vi "SEQUSE~1.VI"(5 "testConfigCluster":T2={"slotIndex"=0, "execMode"=enum."Run", "mainConfigFile"=path "", "criteriaINI"=path "", "totalResult"=FALSE, "stopIfFail"=TRUE, "userControls"={"dialog"=refnum, "testTable"=refnum, "stopButton"=refnum, "statusBox"=refnum}, "testedResult"=enum."DONE", "timeStamp"={"Start"=timestamp(0 s since 1904-01-01), "End"=timestamp(0 s since 1904-01-01)}, "repeatNum"=1, "uutInfo"={"s/n"="", "p/n"="", "productRev"=""}, "sysLanguage"=enum."English", "numOfSocket#"=1, "testRef"="", "testInfo"={"testTime"="", "userID"="", "stationName"="", "testerID"="", "hwVer"="", "swVer"="", "fixtureID"=""}} caption="testConfigCluster (DO NOT REMOVE)", 7 "seqProperties":T1={"Properties"={"processModel"=enum."Single Test", "callSetup"=enum."One-time only when load sequence", "snSetting"={"RequireSnScan?"=TRUE, "digits"=-1.0, "regExp"="", "fixedBarcodeScannerPath"=path ""}, "stopIfFail?"=TRUE, "retestConfirm?"=TRUE, "numTestSocket"=1}, "productInfo"={"Name"="", "Pn"="", "parameter"=variant, "ProdVer"="", "hwVer"="", "swVer"="", "stationName"="", "testerNumber"="1", "fixtureID"=""}, "path"={"criteriaINIPath"=path ""}} caption="seqProperties (DO NOT REMOVE)", 8 "errorIn":errorcluster, 9 "Result?":bool, 11 "sysVar":T4 caption="sysVar (DO NOT REMOVE)") -> (0 "error out":errorcluster, 3 "createLogSuccesful":bool caption="Create Log Succesful (DO NOT REMOVE)")   [LabVIEW 2020]
uses:
  <userlib>/_ATMF/Control_Typedef/__ATMF__SYSTEM__VARIABLE__.ctl
  <userlib>/_ATMF/Control_Typedef/__SEQ__REFERENCE__VARIABLES__.ctl
  <userlib>/_ATMF/Control_Typedef/__SEQ__SYSTEM__CONFIG__UI__USER__DEFINITION__VARIABLES__.ctl
  <userlib>/_ATMF/Tools/Control/__TEST__SEQ__CONFIG__CLUSTER__.ctl
  <userlib>/_ATMF/Control_Typedef/__TEST__STEP__VAR__UI__EXEC__MODE__.ctl
  <userlib>/_ATMF/Control_Typedef/__ATMF__MAIN__TEST__SEQ__PROPERTIES__.ctl
  <vilib>/Comparison/Equal/Equal Functor/Equal Functor.lvclass
panel:
  out "sysVar(Duplicated)":T4
  # "( -1 mean skip check)"
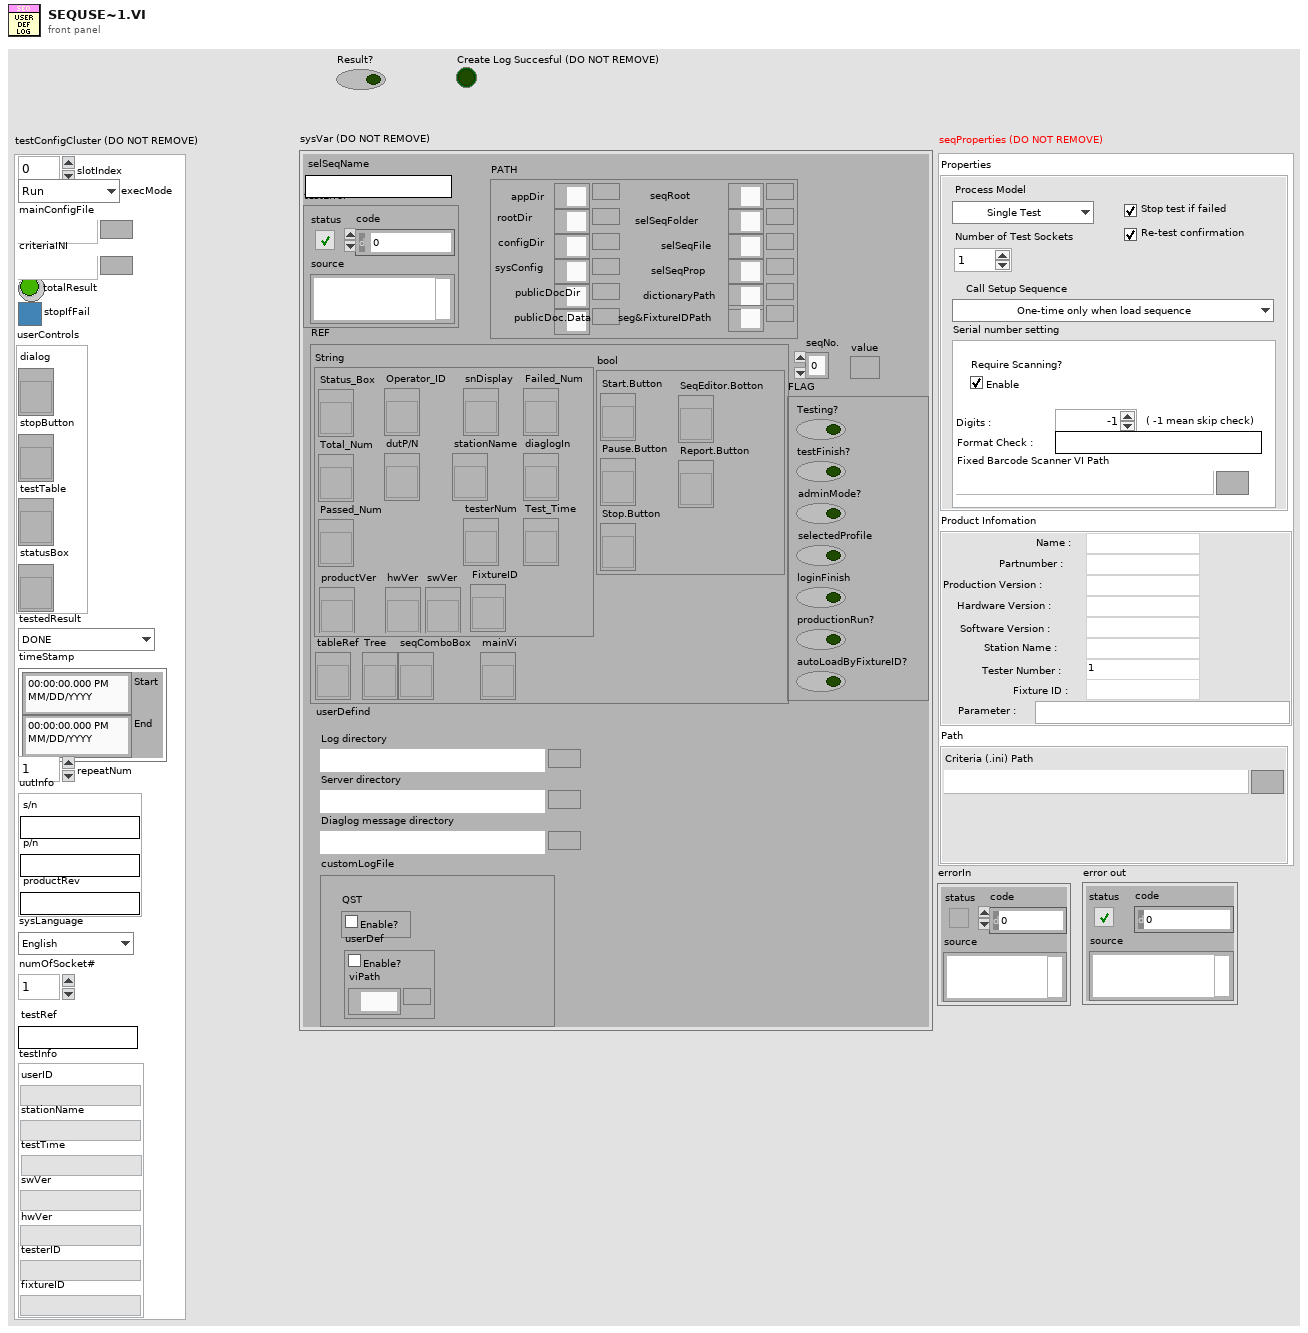
[diagram p1: front panel]
types:
  T1 = typedef "__ATMF__MAIN__TEST__SEQ__PROPERTIES__.ctl" = cluster{"Properties":cluster{"processModel":enum16{"Single Test", "Batch Test", "Parallel Test"}, "callSetup":enum16{"Every test loop", "One-time only when load sequence"}, "snSetting":cluster{"RequireSnScan?":bool, "digits":dbl, "regExp":string, "fixedBarcodeScannerPath":path}, "stopIfFail?":bool, "retestConfirm?":bool, "numTestSocket":u8}, "productInfo":cluster{"Name":string, "Pn":string, "parameter":variant, "ProdVer":string, "hwVer":string, "swVer":string, "stationName":string, "testerNumber":string, "fixtureID":string}, "path":cluster{"criteriaINIPath":path}}
  T2 = typedef "__TEST__SEQ__CONFIG__CLUSTER__.ctl" = cluster{"slotIndex":u8, "execMode":T3, "mainConfigFile":path, "criteriaINI":path, "totalResult":bool, "stopIfFail":bool, "userControls":cluster{"dialog":refnum<vi>, "testTable":refnum<vi>, "stopButton":refnum<vi>, "statusBox":refnum<vi>}, "testedResult":enum16{"DONE", "PASS", "FAIL", "ERROR", "SKIPPED"}, "timeStamp":cluster{"Start":timestamp, "End":timestamp}, "repeatNum":u8, "uutInfo":cluster{"s/n":string, "p/n":string, "productRev":string}, "sysLanguage":enum16{"English", "Chinese", "Thai"}, "numOfSocket#":u8, "testRef":string, "testInfo":cluster{"testTime":string, "userID":string, "stationName":string, "testerID":string, "hwVer":string, "swVer":string, "fixtureID":string}}
  T3 = typedef "__TEST__STEP__VAR__UI__EXEC__MODE__.ctl" = enum16{"Run", "Debug", "Edit", "Open VI"}
  T4 = typedef "__ATMF__SYSTEM__VARIABLE__.ctl" = cluster{"seqNo.":i32, "testError":errorcluster, "value":variant, "REF":T5, "PATH":cluster{"appDir":path, "rootDir":path, "configDir":path, "sysConfig":path, "publicDocDir":path, "publicDoc.Data":path, "seqRoot":path, "selSeqFolder":path, "selSeqFile":path, "selSeqProp":path, "dictionaryPath":path, "seg&FixtureIDPath":path}, "FLAG":cluster{"Testing?":bool, "testFinish?":bool, "adminMode?":bool, "selectedProfile":bool, "loginFinish":bool, "productionRun?":bool, "autoLoadByFixtureID?":bool}, "userDefind":T6, "selSeqName":string, "customLogFile":cluster{"QST":cluster{"Enable?":bool}, "userDef":cluster{"Enable?":bool, "viPath":path}}}
  T5 = typedef "__SEQ__REFERENCE__VARIABLES__.ctl" = cluster{"String":cluster{"Status_Box":refnum<vi>, "Total_Num":refnum<vi>, "Passed_Num":refnum<vi>, "Failed_Num":refnum<vi>, "diaglogIn":refnum<vi>, "Test_Time":refnum<vi>, "Operator_ID":refnum<vi>, "snDisplay":refnum<vi>, "stationName":refnum<vi>, "testerNum":refnum<vi>, "productVer":refnum<vi>, "dutP/N":refnum<vi>, "hwVer":refnum<vi>, "swVer":refnum<vi>, "FixtureID":refnum<vi>}, "bool":cluster{"SeqEditor.Botton":refnum<vi>, "Start.Button":refnum<vi>, "Pause.Button":refnum<vi>, "Stop.Button":refnum<vi>, "Report.Button":refnum<vi>}, "tableRef":refnum<vi>, "Tree":refnum<vi>, "seqComboBox":refnum<vi>, "mainVi":refnum<vi>}
  T6 = typedef "__SEQ__SYSTEM__CONFIG__UI__USER__DEFINITION__VARIABLES__.ctl" = cluster{"resultLog":path, "serverLogPath":path, "diagMsgDir":path}
  T7 = cluster{"resultArray2D[]":string[][], "createLogSuccesful":bool}
  T8 = enum16{"Reset", "Yellow Lamp&Alarm", "Green Lamp&Alarm", "Red Lamp&Alarm"}
  T9 = enum16{"Step", "Description", "Min", "Measure", "Max", "Unit", "Status"}
  T10 = enum16{"open", "replace", "create", "open or create", "replace or create", "replace or create with confirmation"}
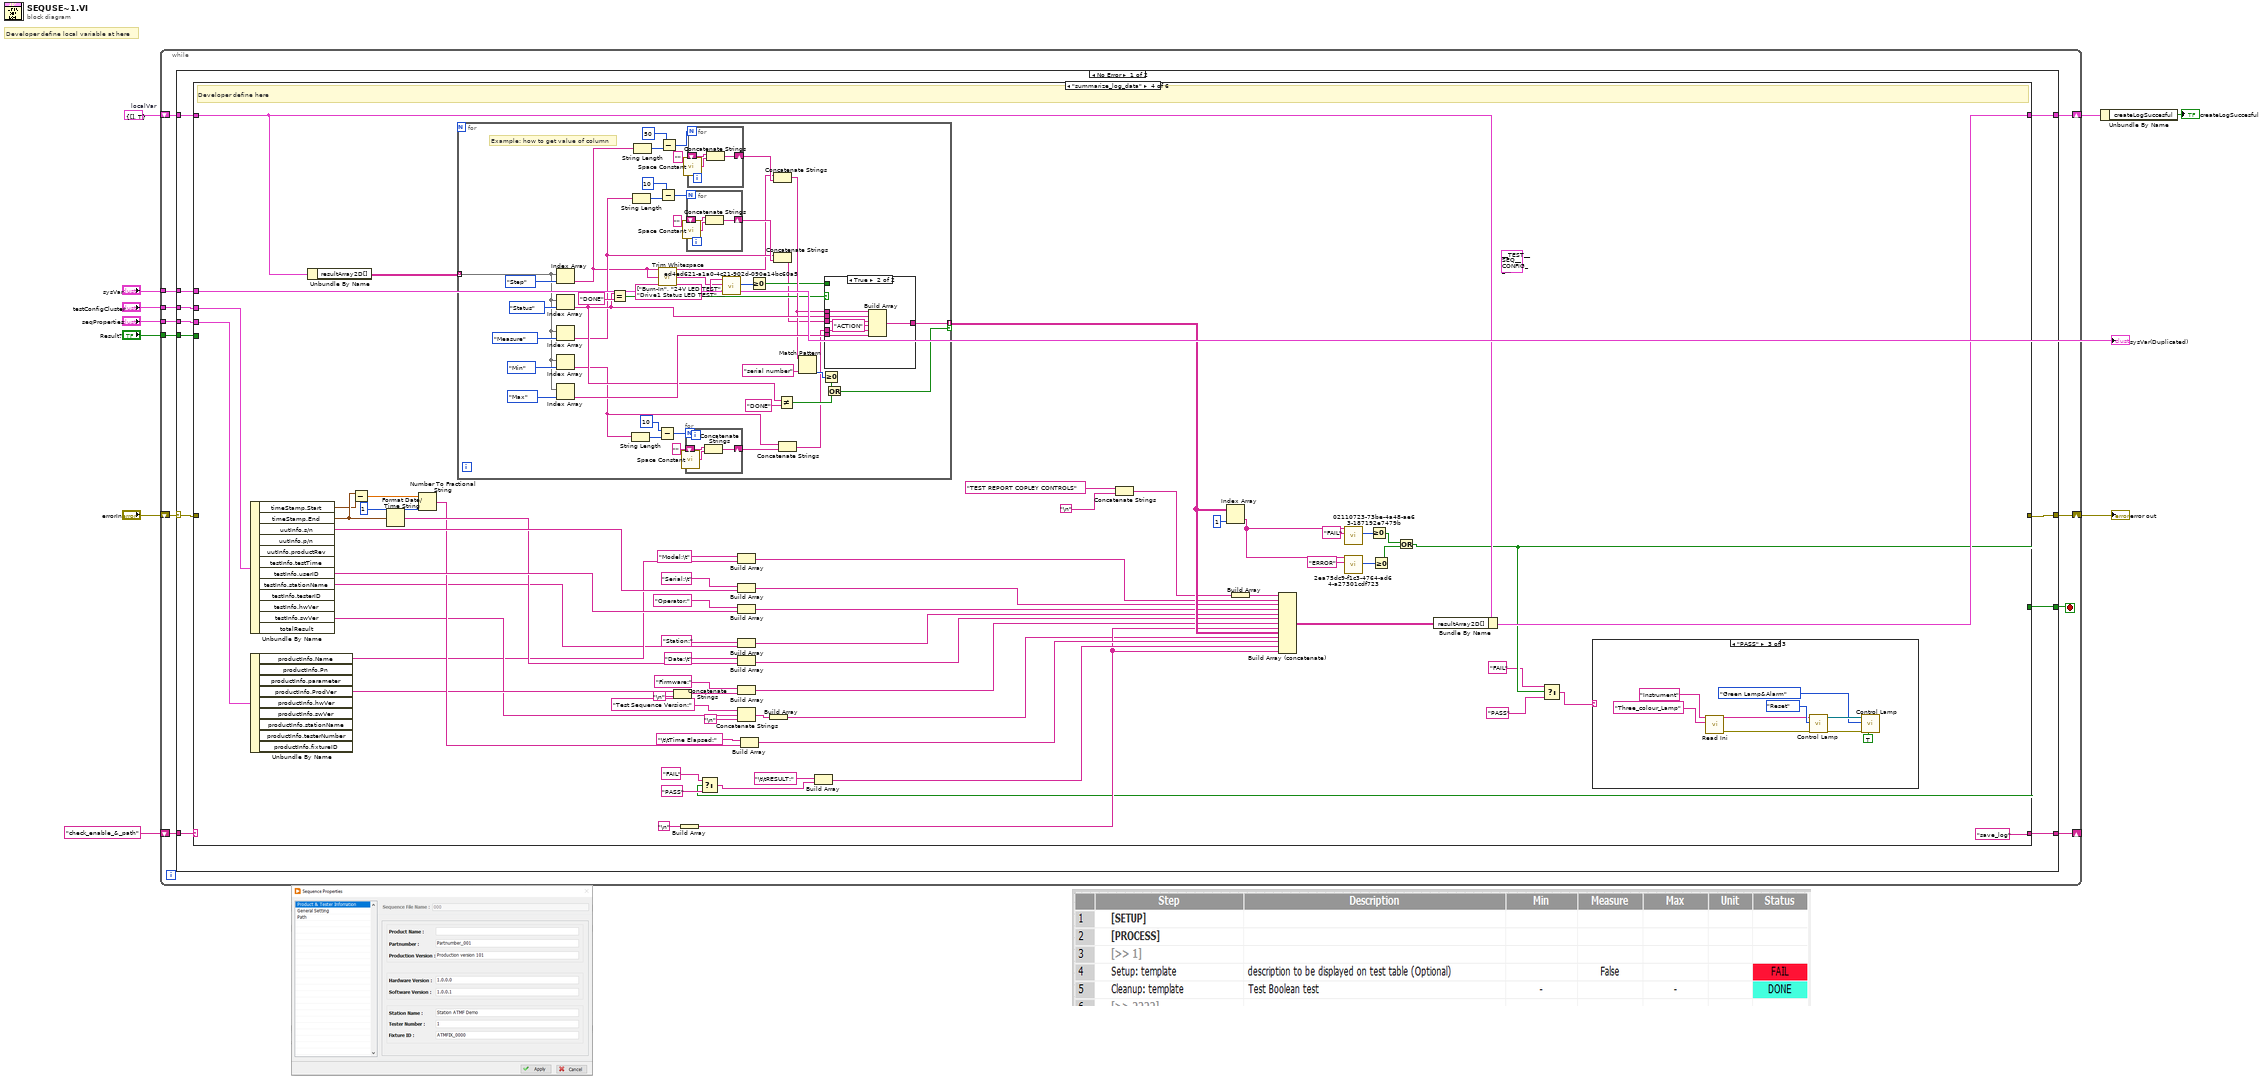
[diagram p0: block diagram]
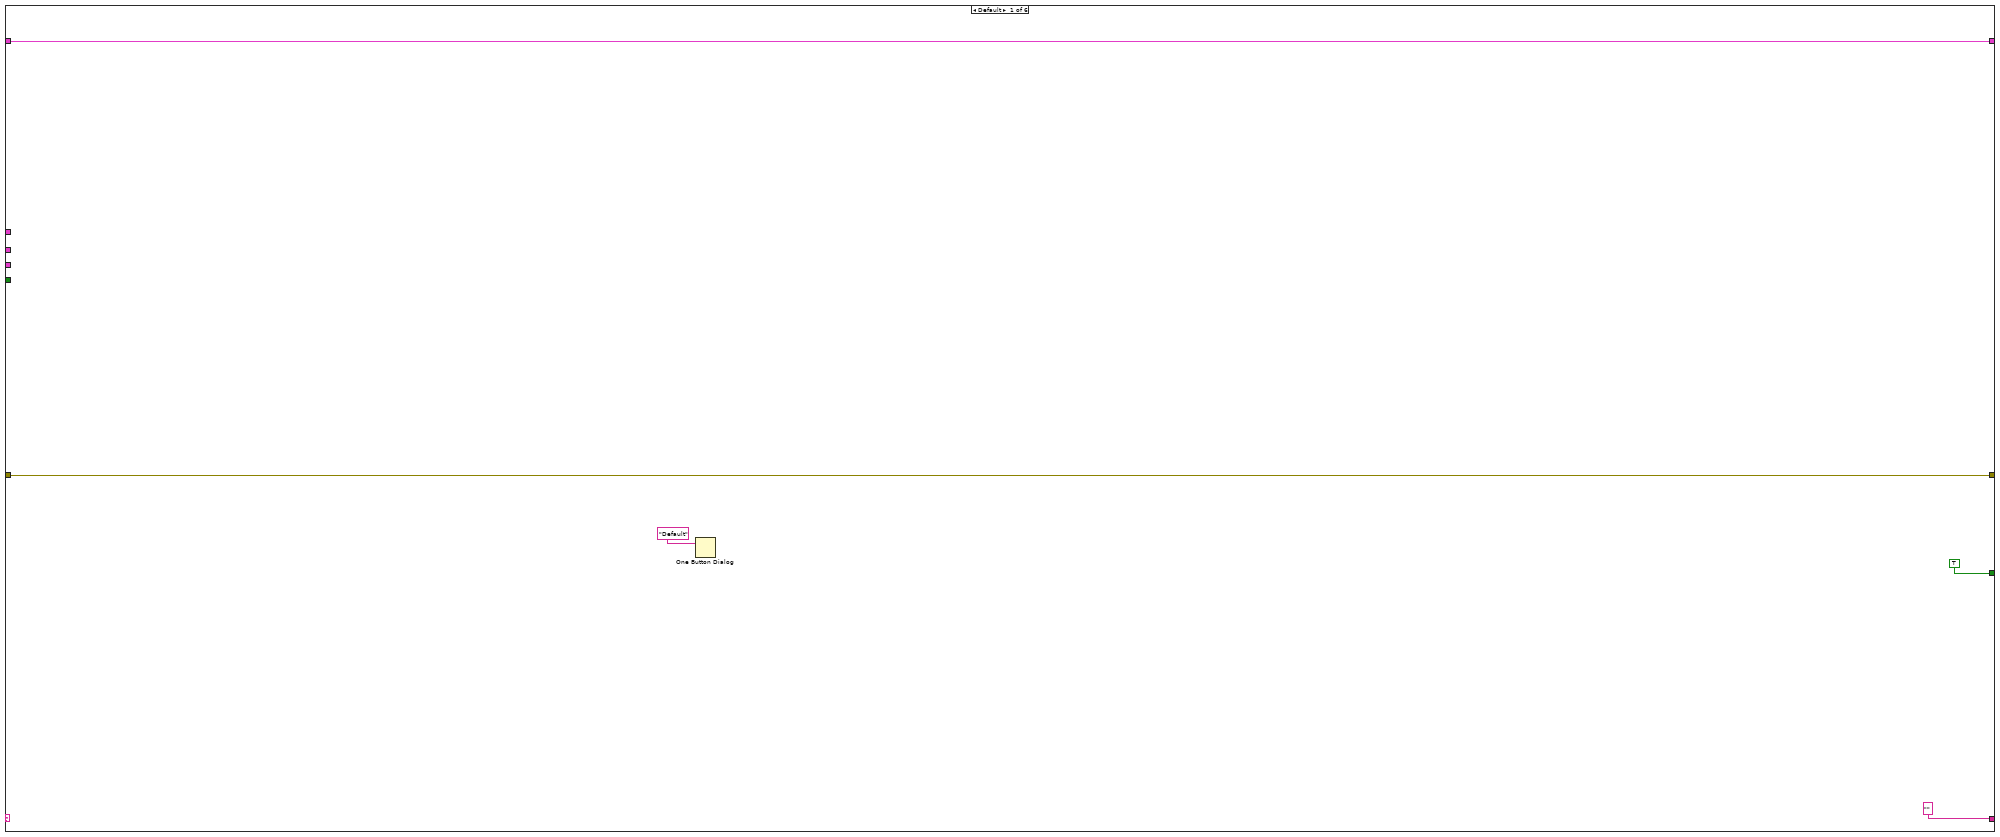
[diagram p2: hidden frame]
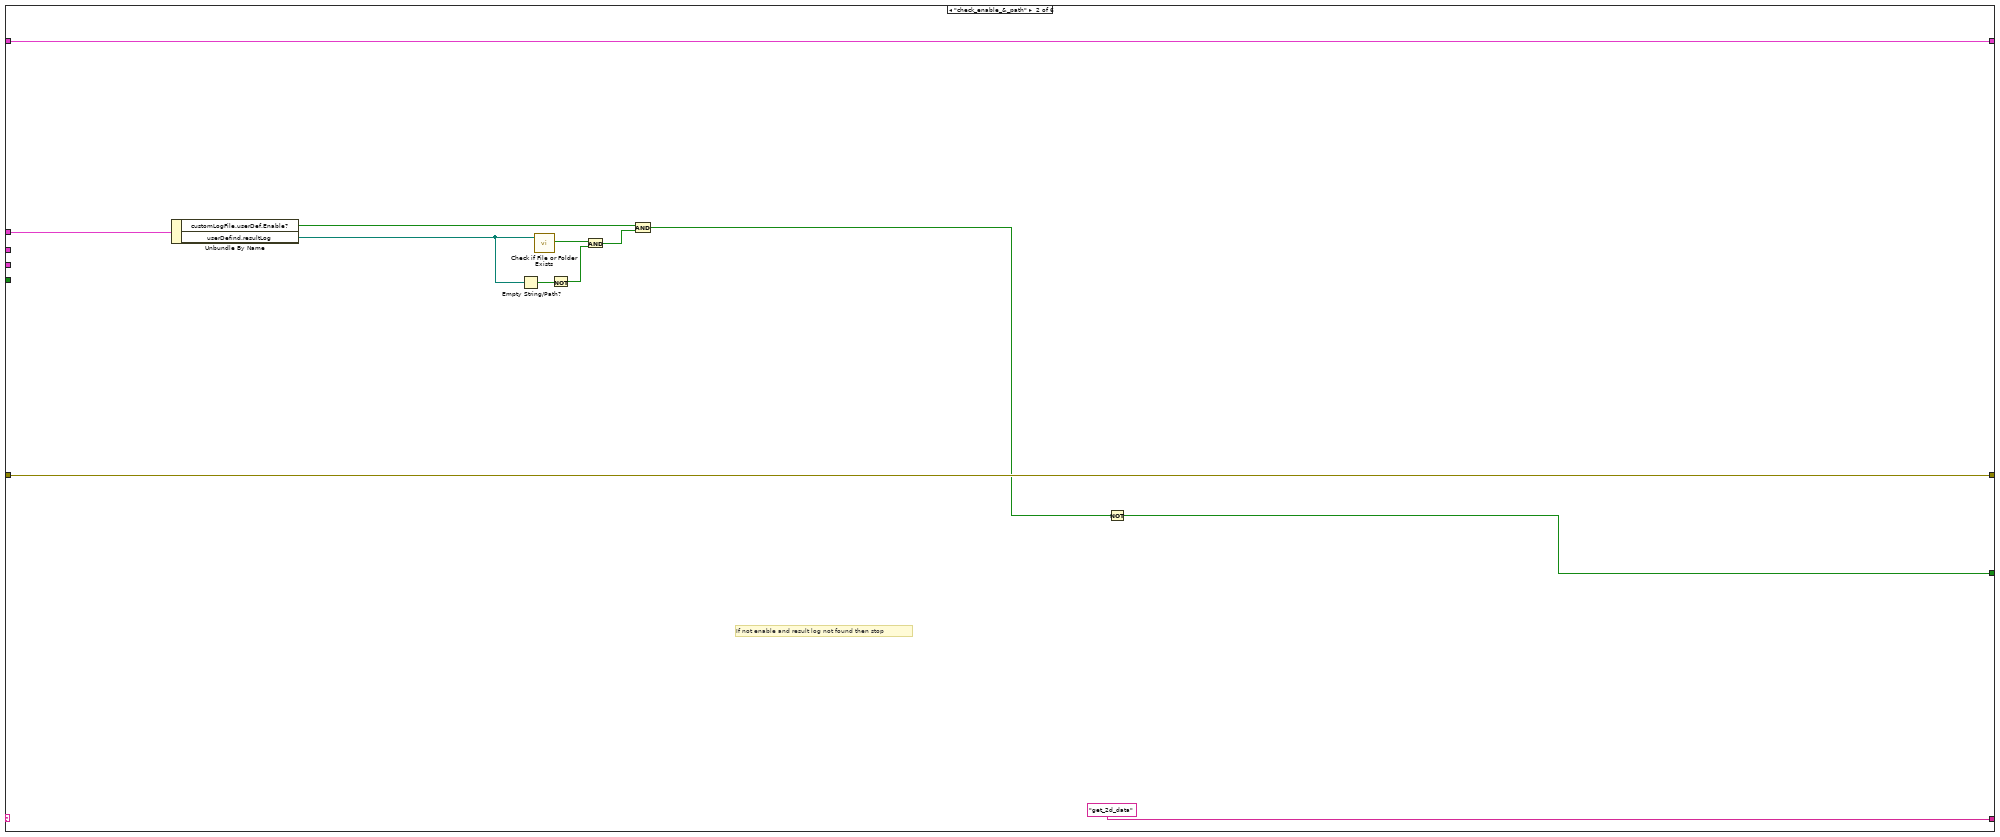
[diagram p3: hidden frame]
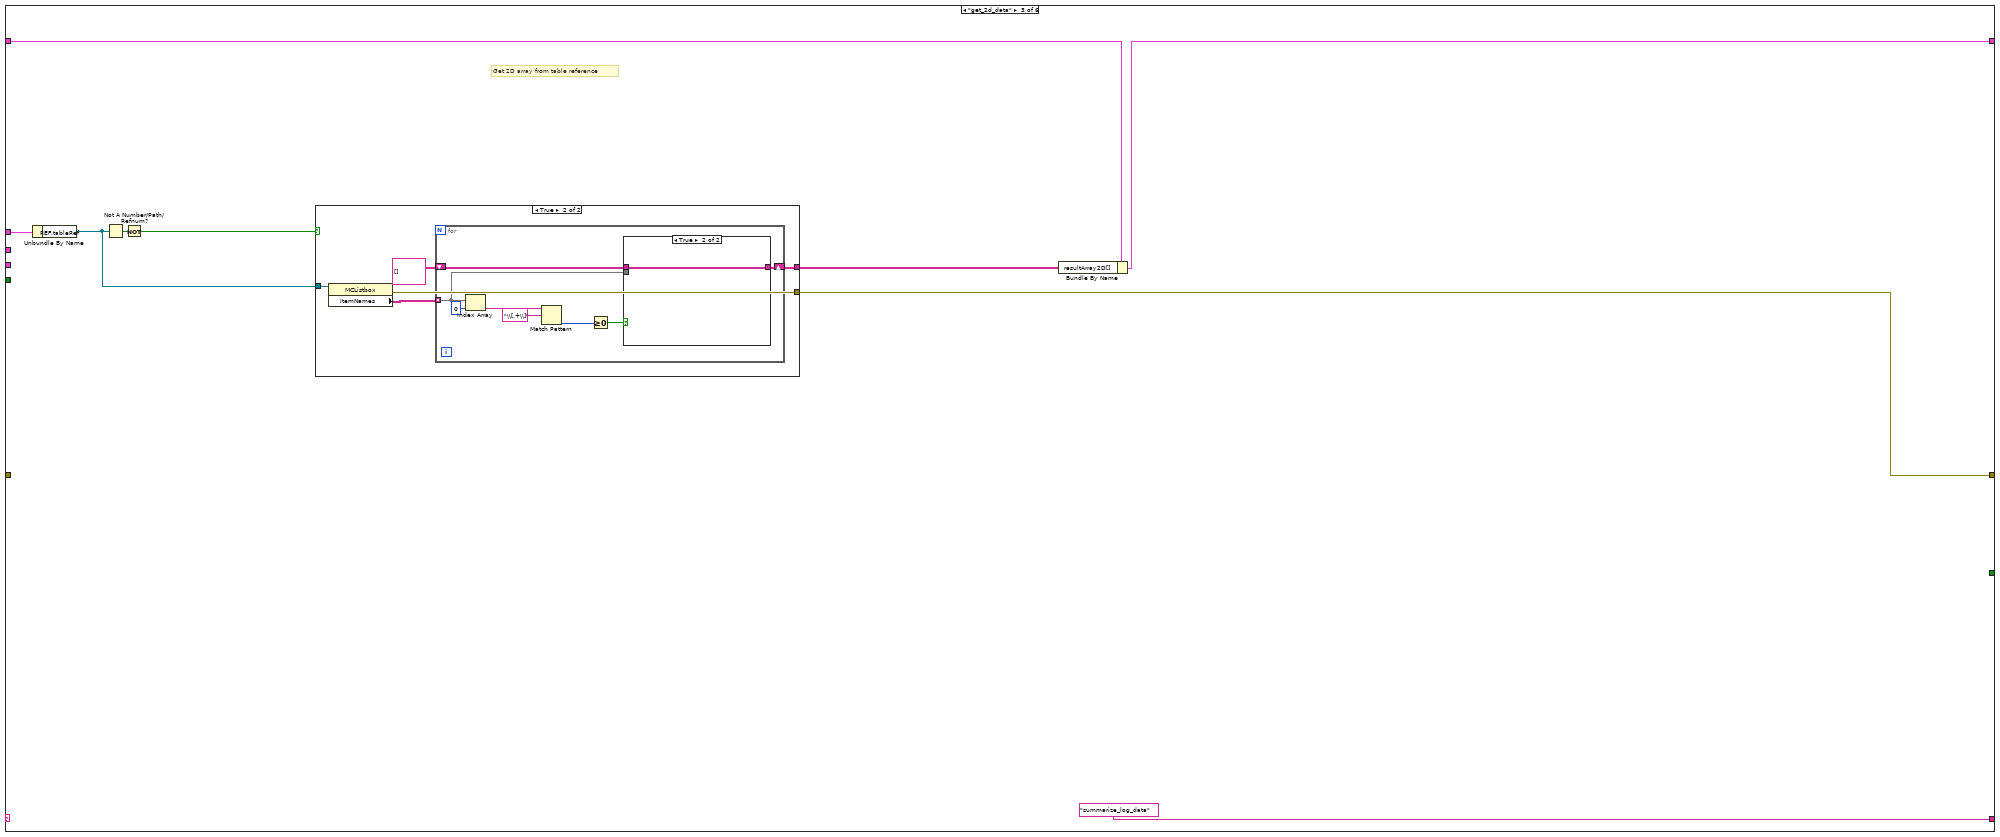
[diagram p4: hidden frame]
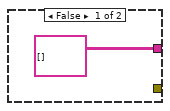
[diagram p5: hidden frame]
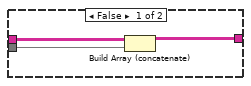
[diagram p6: hidden frame]
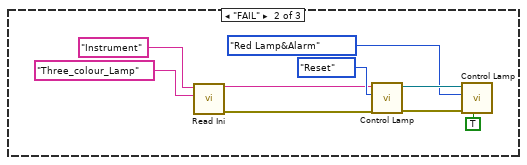
[diagram p8: hidden frame]
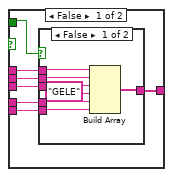
[diagram p9: hidden frame]
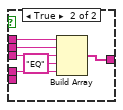
[diagram p10: hidden frame]
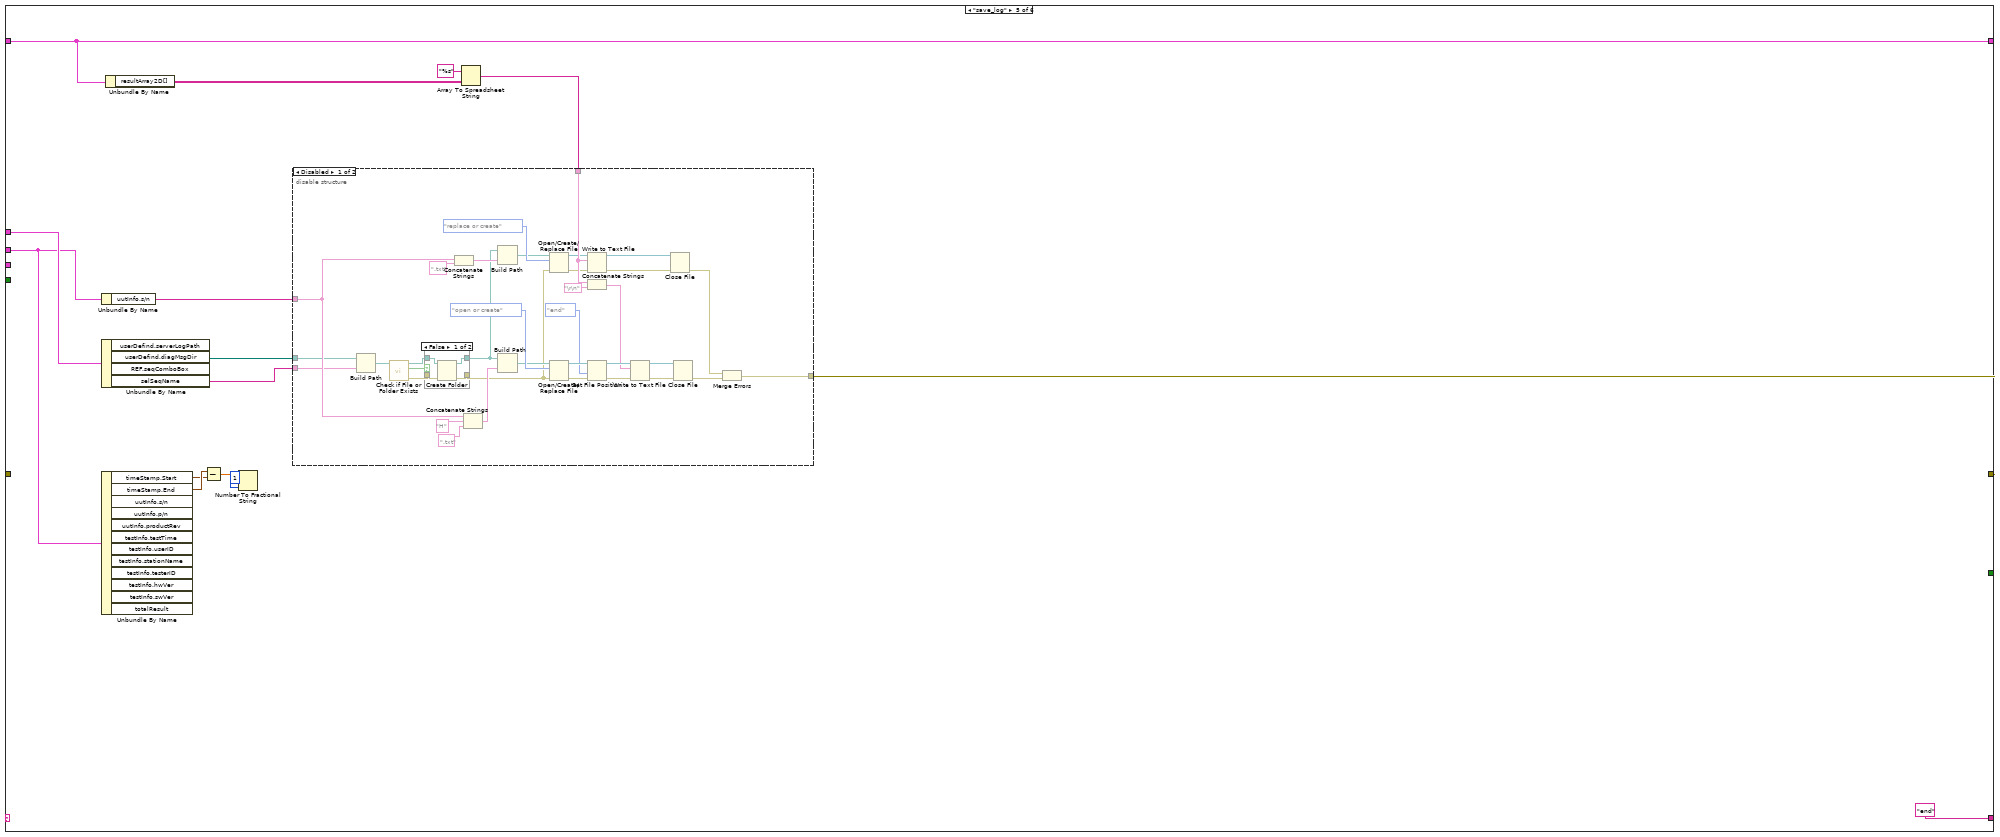
[diagram p11: hidden frame]
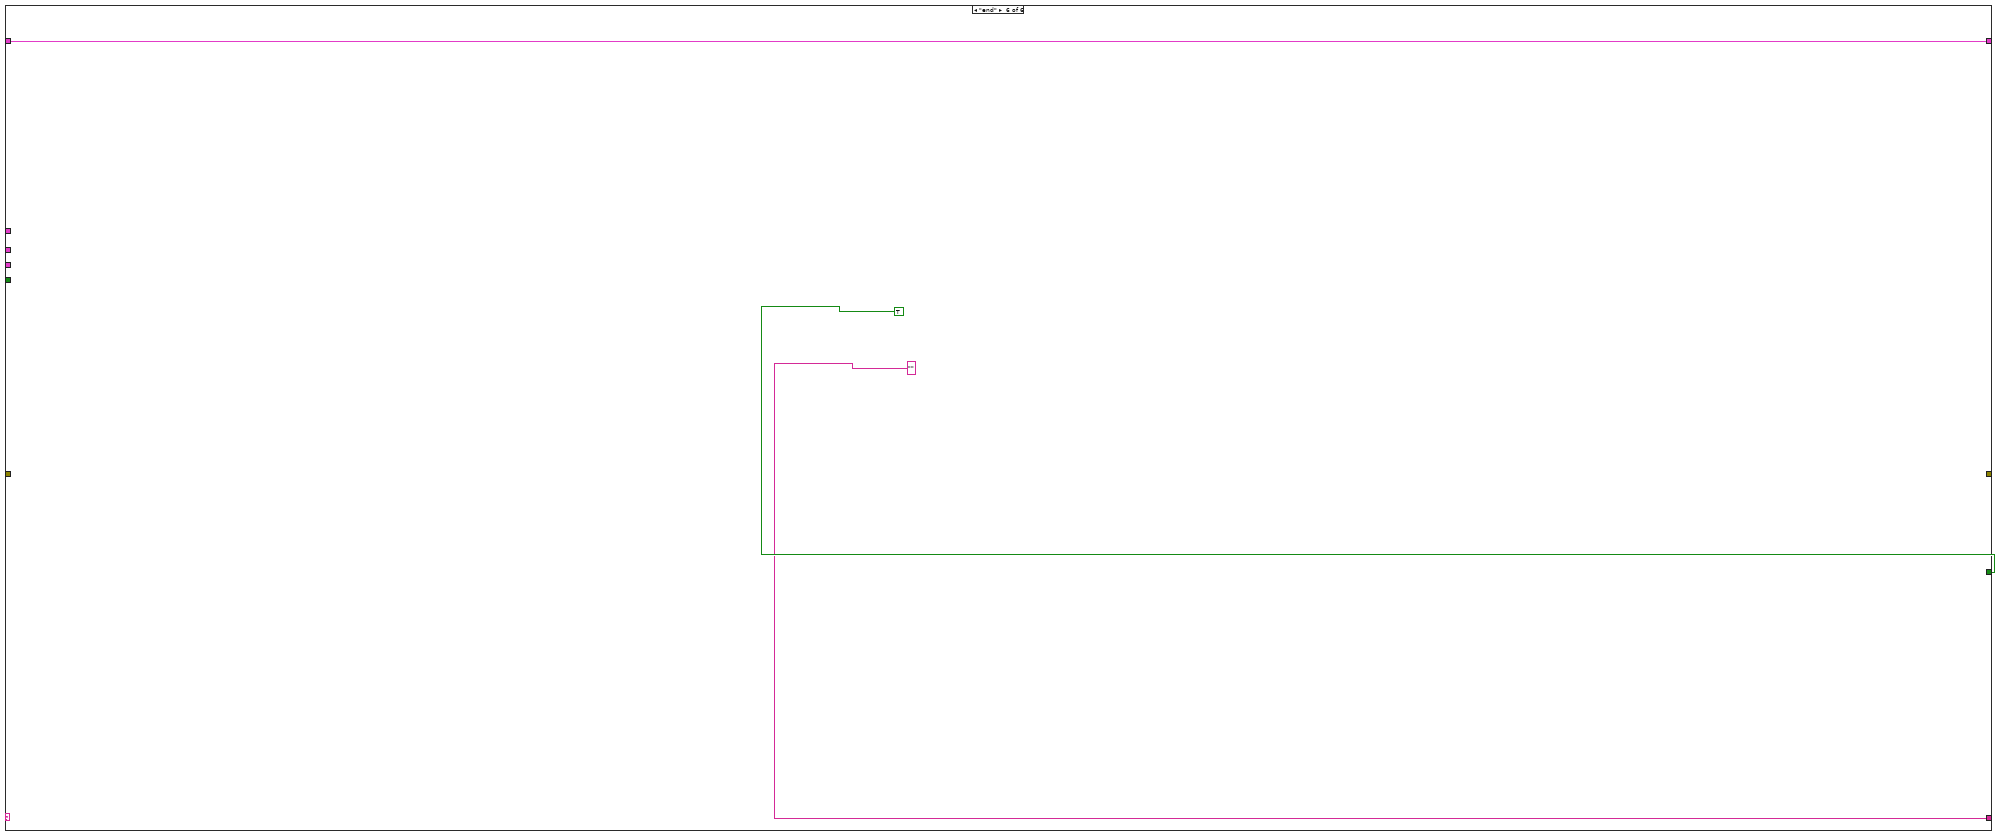
[diagram p14: hidden frame]
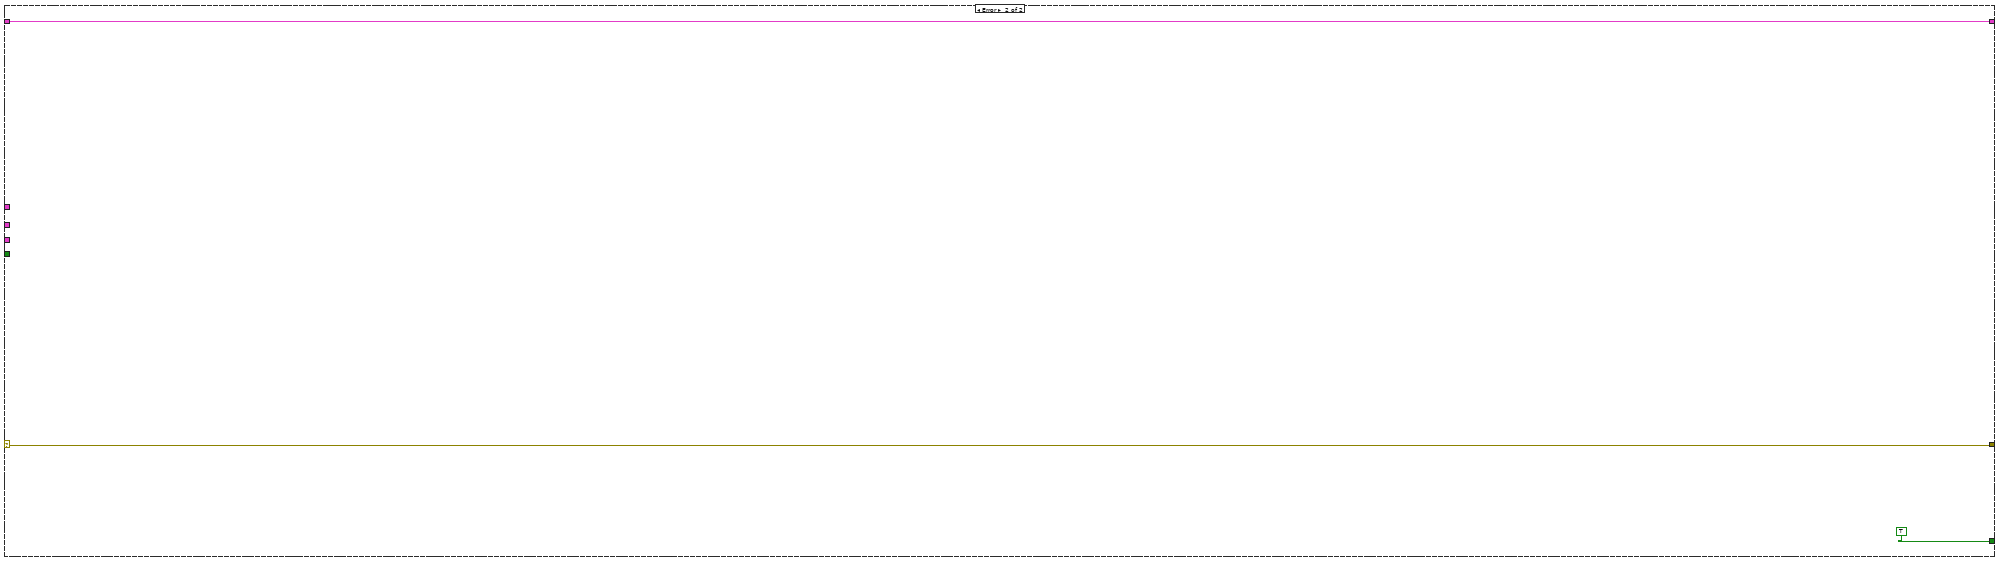
[diagram p15: hidden frame]
diagram:
  w3 = T7 {"resultArray2D[]"=[], "createLogSuccesful"=TRUE}  # localVar
  # "Developer define local variable at here"
  n1 = while {
    shift-right: [w19] -> w10
    shift-left: "errorIn" -> [w20]
    tunnel: "sysVar" -> [w17]
    tunnel: "testConfigCluster" -> [w16]
    tunnel: "seqProperties" -> [w15]
    shift-right: [w18] -> _
    shift-left: "check_enable_&_path" -> [w21]
    tunnel: "Result?" -> [w14]
    shift-right: [w11] -> w2
    shift-left: w3 -> [w12]
    stop <- w13 stop-if-true
    n2 = case shown="No Error" w20 {
      selector: w20 -> [w31 w297]
      tunnel: w21 -> [w32 _]
      tunnel: [w30 w297] -> w19
      tunnel: [w29 _] -> w18
      tunnel: w17 -> [w28 _]
      tunnel: w16 -> [w27 _]
      tunnel: w15 -> [w26 _]
      tunnel: w14 -> [w25 _]
      tunnel: [w24 TRUE] -> w13
      tunnel: w12 -> [w23 w295]
      tunnel: [w22 w295] -> w11
      frame No Error {
        n3 = case shown="\"summarize_log_data\"" w32 {
          tunnel: w31 -> [w37 w49 _ _ _ _]
          tunnel: [w37 w49 w50 _ w246 _] -> w30
          tunnel: ["" "get_2d_data" "summarize_log_data" "save_log" "end" ""] -> w29
          tunnel: w28 -> [_ w41 w58 _ w242 _]
          tunnel: w27 -> [_ _ _ w85 w236 _]
          tunnel: w26 -> [_ _ _ w88 _ _]
          tunnel: w25 -> [_ _ _ _ _ _]
          tunnel: [TRUE w39 _ _ _ TRUE] -> w24
          tunnel: w23 -> [w34 w38 w54 w138 w249 w294]
          tunnel: [w34 w38 w53 w92 w249 w294] -> w22
          frame Default {
            n4 = One Button Dialog(message="Default") -> ()  [unwired: 1 in, 1 out]
          }
          frame "check_enable_&_path" {
            # "If not enable and result log not found then stop"
            n5 = Unbundle By Name(w41) -> ("customLogFile.userDef.Enable?"=w42:bool, "userDefind.resultLog"=w46:path)
            n6 = Empty String/Path?(string/path=w46) -> (empty?=w43:bool)
            n7 = call <vilib>:"Check if File or Folder Exists.vi"("path"=w46) -> ("file or folder exists?"=w44:bool)  [unwired: 8 in, 2 out]
            n8 = Not(x=w43) -> (.not. x?=w45:bool)
            n9 = And(x=w44, y=w45) -> (x .and. y?=w47:bool)
            n10 = And(x=w42, y=w47) -> (x .and. y?=w40:bool)
            n11 = Not(x=w40) -> (.not. x?=w39:bool)
          }
          frame "get_2d_data" {
            # "Get 2D array from table reference"
            n12 = Unbundle By Name(w58) -> ("REF.tableRef"=w55:refnum<vi>)
            n13 = Not A Number/Path/Refnum?(number/path/refnum=w55) -> (NaN/Path/Refnum?=w57:bool)
            n14 = Not(x=w57) -> (.not. x?=w56:bool)
            n15 = case shown="True" w56 {
              tunnel: [string[][] [] w62] -> w52
              tunnel: w55 -> [_ w61]
              tunnel: [_ w60] -> w50
              frame False {
              }
              frame True {
                n16 = property class="MCListbox"(reference=w61) -> (error out=w60:errorcluster, "ItemNames"=w64:string[][])  [unwired: 1 in, 1 out]
                n17 = for {
                  tunnel: w64 -> [w65] mode=indexing
                  shift-right: [w68] -> w62
                  shift-left: string[][] [] -> [w69]
                  n18 = Index Array(array=w65, index=0) -> (element=w71:string)
                  n19 = Match Pattern(string=w71, regular expression="\\[.+\\]") -> (offset past match=w67:i32)  [unwired: 1 in, 3 out]
                  n20 = Greater Or Equal To 0?(x=w67) -> (x >= 0?=w66:bool)
                  n21 = case shown="True" w66 {
                    tunnel: w69 -> [w75 w76]
                    tunnel: [w74 w76] -> w68
                    tunnel: w65 -> [w73 _]
                    frame False {
                      n22 = Build Array (concatenate)(w75, w73) -> (w74:string[][])
                    }
                    frame True {
                    }
                  }
                }
              }
            }
            n23 = Bundle By Name(cluster=w54, "resultArray2D[]"=w52) -> (w53:T7)
          }
          frame "summarize_log_data" {
            (unwired) T2 {"slotIndex"=0, "execMode"=enum."Run", "mainConfigFile"=path "", "criteriaINI"=path "", "totalResult"=FALSE, "stopIfFail"=FALSE, "userControls"={"dialog"=refnum, "testTable"=refnum, "stopButton"=refnum, "statusBox"=refnum}, "testedResult"=enum."DONE", "timeStamp"={"Start"=timestamp(0 s since 1904-01-01), "End"=timestamp(0 s since 1904-01-01)}, "repeatNum"=1, "uutInfo"={"s/n"="", "p/n"="", "productRev"=""}, "sysLanguage"=enum."English", "numOfSocket#"=1, "testRef"="", "testInfo"={"testTime"="", "userID"="", "stationName"="", "testerID"="", "hwVer"="", "swVer"="", "fixtureID"=""}} ("testConfigCluster")
            # "Developer define here"
            n24 = Unbundle By Name(w85) -> ("timeStamp.Start"=w120:timestamp, "timeStamp.End"=w121:timestamp, "uutInfo.s/n"=w135:string, "testInfo.userID"=w133:string, "testInfo.stationName"=w83:string, "testInfo.swVer"=w94:string)  [unwired: 6 out]
            n25 = Unbundle By Name(w88) -> ("productInfo.Name"=w84:string, "productInfo.ProdVer"=w98:string)  [unwired: 7 out]
            n26 = Unbundle By Name(w138) -> ("resultArray2D[]"=w86:string[][])
            n27 = Subtract(x=w121, y=w120) -> (x-y=w119:dbl)
            n28 = Format Date/Time String(seconds (now)=w121) -> (date/time string=w130:string)  [unwired: 2 in]
            n29 = Number To Fractional String(number=w119, precision (6)=i16 1) -> (F-format string=w117:string)  [unwired: 2 in]
            n30 = for {
              tunnel: w86 -> [w179] mode=indexing
              tunnel: [w193] -> w116 mode=indexing if=w186
              # "Example: how to get value of column"
              n31 = Index Array(array=w179, index=T9."Step") -> (element=w166:string)
              n32 = Index Array(array=w179, index=T9."Status") -> (element=w185:string)
              n33 = Index Array(array=w179, index=T9."Measure") -> (element=w169:string)
              n34 = Index Array(array=w179, index=T9."Min") -> (element=w159:string)
              n35 = Index Array(array=w179, index=T9."Max") -> (element=w194:string)
              n36 = Equal?(x=w185, y="DONE") -> (x = y?=w176:bool)
              n37 = String Length(string=w159) -> (length=w162:i32)
              n38 = String Length(string=w169) -> (length=w171:i32)
              n39 = String Length(string=w166) -> (length=w184:i32)
              n40 = Subtract(x=10, y=w162) -> (x-y=w163:i32)
              n41 = call <vilib>:"Trim Whitespace.vi"("string"=w166) -> ("trimmed string"=w165:string)  [unwired: 1 in]
              n42 = Subtract(x=10, y=w171) -> (x-y=w173:i32)
              n43 = Subtract(x=50, y=w184) -> (x-y=w182:i32)
              n44 = for {
                N: w163 -> [_]
                shift-right: [w202] -> w160
                shift-left: "" -> [w201]
                n45 = call <vilib>:"Space Constant.vi"() -> ("String"=w200:string)
                n46 = Concatenate Strings(w201, w200) -> (w202:string)
              }
              n47 = for {
                N: w173 -> [_]
                shift-right: [w205] -> w170
                shift-left: "" -> [w204]
                n48 = call <vilib>:"Space Constant.vi"() -> ("String"=w203:string)
                n49 = Concatenate Strings(w204, w203) -> (w205:string)
              }
              n50 = for {
                N: w182 -> [_]
                shift-right: [w235] -> w180
                shift-left: "" -> [w234]
                n51 = call <vilib>:"Space Constant.vi"() -> ("String"=w233:string)
                n52 = Concatenate Strings(w234, w233) -> (w235:string)
              }
              n53 = call "ed4ed621-a1a0-4c21-902d-090e14bc60a5.vi"("element"=w165, "unsorted 1D array"=string[] ["Burn-In", "24V LED TEST", "Drive1 Status LED TEST", "Drive2 Status LED TEST", "Drive3 Status LED TEST", "Fan1 Test", "Fan2 Test", "Fan3 Test", "Get drive1 serial number", "Get drive2 serial number", "Get drive3 serial number", "Drive1 model number check", "Drive2 model number check", "Drive3 model number check", "Drive1 firmware version check", "Drive2 firmware version check", "Drive3 firmware version check", "Fault1 Monitor_Coil1_AMPPROG1_0V", "Fault1 Monitor_Coil1_AMPPROG1_2.5V", "Fault1 Monitor_Coil1_AMPPROG1_5V", "LED Test_the fault of M1 drive", "Fault1 Monitor_M1 Drive Fault Signal", "LED Test_Reset Drive", "Fault1 Monitor_Reset Drive", "Fault2 Monitor_Coil2_AMPPROG2_0V", "Fault2 Monitor_Coil2_AMPPROG2_2.5V", "Fault2 Monitor_Coil2_AMPPROG2_5V", "LED Test_the fault of M1 drive", "Fault2 Monitor_M1 Drive Fault Signal", "LED Test_Reset Drive", "Fault2 Monitor_Reset Drive", "Fault3 Monitor_Coil3_AMPPROG3_0V", "Fault3 Monitor_Coil3_AMPPROG3_2.5V", "Fault3 Monitor_Coil3_AMPPROG3_5V", "LED Test_the fault of M1 drive", "Fault3 Monitor_M1 Drive Fault Signal", "LED Test_Reset Drive", "Fault3 Monitor_Reset Drive", "Fault4 Monitor_Coil4_AMPPROG4_0V", "Fault4 Monitor_Coil4_AMPPROG4_2.5V", "Fault4 Monitor_Coil4_AMPPROG4_5V", "LED Test_the fault of M1 drive", "Fault4 Monitor_M1 Drive Fault Signal", "LED Test_Reset Drive", "Fault4 Monitor_Reset Drive", "Fault5 Monitor_Coil5_AMPPROG5_0V", "Fault5 Monitor_Coil5_AMPPROG5_2.5V", "Fault5 Monitor_Coil5_AMPPROG5_5V", "LED Test_the fault of M2 drive", "Fault5 Monitor_M2 Drive Fault Signal", "LED Test_Reset Drive", "Fault5 Monitor_Reset Drive", "Fault6 Monitor_Coil6_AMPPROG6_0V", "Fault6 Monitor_Coil6_AMPPROG6_2.5V", "Fault6 Monitor_Coil6_AMPPROG6_5V", "LED Test_the fault of M2 drive", "Fault6 Monitor_M2 Drive Fault Signal", "LED Test_Reset Drive", "Fault6 Monitor_Reset Drive", "Fault7 Monitor_Coil7_AMPPROG7_0V", "Fault7 Monitor_Coil7_AMPPROG7_2.5V", "Fault7 Monitor_Coil7_AMPPROG7_5V", "LED Test_the fault of M2 drive", "Fault7 Monitor_M2 Drive Fault Signal", "LED Test_Reset Drive", "Fault7 Monitor_Reset Drive", "Fault8 Monitor_Coil8_AMPPROG8_0V", "Fault8 Monitor_Coil8_AMPPROG8_2.5V", "Fault8 Monitor_Coil8_AMPPROG8_5V", "LED Test_the fault of M2 drive", "Fault8 Monitor_M2 Drive Fault Signal", "LED Test_Reset Drive", "Fault8 Monitor_Reset Drive", "Fault9 Monitor_Coil9_AMPPROG9_0V", "Fault9 Monitor_Coil9_AMPPROG9_2.5V", "Fault9 Monitor_Coil9_AMPPROG9_5V", "LED Test_the fault of M3 drive", "Fault9 Monitor_M3 Drive Fault Signal", "LED Test_Reset Drive", "Fault9 Monitor_Reset Drive", "Fault10 Monitor_Coil10_AMPPROG10_0V", "Fault10 Monitor_Coil10_AMPPROG10_2.5V", "Fault10 Monitor_Coil10_AMPPROG10_5V", "LED Test_the fault of M3 drive", "Fault10 Monitor_M3 Drive Fault Signal", "LED Test_Reset Drive", "Fault10 Monitor_Reset Drive", "Fault11 Monitor_Coil11_AMPPROG11_0V", "Fault11 Monitor_Coil11_AMPPROG11_2.5V", "Fault11 Monitor_Coil11_AMPPROG11_5V", "LED Test_the fault of M3 drive", "Fault11 Monitor_M3 Drive Fault Signal", "LED Test_Reset Drive", "Fault11 Monitor_Reset Drive", "Get drive1 serial number", "Get drive2 serial number", "Get drive3 serial number", "Drive1 model number check", "Drive2 model number check", "Drive3 model number check", "Drive1 firmware version check", "Drive2 firmware version check", "Drive3 firmware version check", "Cleanup: Power OFF", "", "", "", "", "", ""] ("Array")) -> ("index of element"=w177:i32)  [unwired: 9 in]
              n54 = Greater Or Equal To 0?(x=w177) -> (x >= 0?=w175:bool)
              n55 = Concatenate Strings(w166, w180) -> (w181:string)
              n56 = Concatenate Strings(w169, w170) -> (w168:string)
              n57 = Not Equal?(x=w185, y="DONE") -> (x != y?=w187:bool)
              n58 = Concatenate Strings(w159, w160) -> (w158:string)
              n59 = Match Pattern(string=w181, regular expression="serial number") -> (offset past match=w189:i32)  [unwired: 1 in, 3 out]
              n60 = Greater Or Equal To 0?(x=w189) -> (x >= 0?=w188:bool)
              n61 = case shown="True" w176 {
                tunnel: w168 -> [w210 w232]
                tunnel: w158 -> [w209 w231]
                tunnel: w194 -> [w208 w230]
                tunnel: [w207 w229] -> w193
                tunnel: w185 -> [w211 w228]
                tunnel: w181 -> [w212 w227]
                tunnel: w175 -> [w206 _]
                frame False {
                  n62 = case shown="False" w206 {
                    tunnel: w212 -> [w219 w225]
                    tunnel: w211 -> [w218 w224]
                    tunnel: w210 -> [w217 w223]
                    tunnel: w209 -> [w216 w222]
                    tunnel: w208 -> [w215 _]
                    tunnel: [w213 w221] -> w207
                    frame False {
                      n63 = Build Array(w219, w218, w217, "GELE" ("element"), w216, w215) -> (w213:string[])
                    }
                    frame True {
                      n64 = Build Array(w225, w224, w223, "EQ" ("element"), w222) -> (w221:string[])
                    }
                  }
                }
                frame True {
                  n65 = Build Array(w227, w228, w232, "ACTION" ("element"), w231, w230) -> (w229:string[])
                }
              }
              n66 = Or(x=w188, y=w187) -> (x .or. y?=w186:bool)
            }
            n67 = Concatenate Strings(w98, "\n") -> (w97:string)
            n68 = Build Array("\n") -> (w102:string[])
            n69 = Build Array("Model:\t" ("string"), w84) -> (w105:string[])
            n70 = Build Array("Serial:\t" ("string"), w135) -> (w104:string[])
            n71 = Build Array("Operator:" ("string"), w133) -> (w87:string[])
            n72 = Build Array("Station:" ("string"), w83) -> (w89:string[])
            n73 = Build Array("Date:\t" ("string"), w130) -> (w103:string[])
            n74 = Build Array("Firmware:" ("element"), w97) -> (w81:string[])
            n75 = Concatenate Strings("Test Sequence Version:" ("string"), w94, "\n") -> (w95:string)
            n76 = Build Array("\t\tTime Elapsed:", w117) -> (w123:string[])
            n77 = Build Array(w95) -> (w90:string[])
            n78 = Concatenate Strings("TEST REPORT COPLEY CONTROLS", "\n") -> (w99:string)
            n79 = Index Array(array=w116, index (col)=1 ("disabled index (col)")) -> (element=w113:string[])  [unwired: 1 in]
            n80 = Build Array(w99) -> (w107:string[])
            n81 = call "02110723-73be-4a48-ae63-187192e7479b.vi"("element"="FAIL", "unsorted 1D array"=w113) -> ("index of element"=w111:i32)  [unwired: 9 in]
            n82 = call "2ea75dc9-f1c3-4764-ad64-a27301cdf723.vi"("element"="ERROR", "unsorted 1D array"=w113) -> ("index of element"=w110:i32)  [unwired: 9 in]
            n83 = Greater Or Equal To 0?(x=w111) -> (x >= 0?=w109:bool)
            n84 = Greater Or Equal To 0?(x=w110) -> (x >= 0?=w108:bool)
            n85 = Or(x=w109, y=w108) -> (x .or. y?=w80:bool)
            n86 = Select(t="FAIL", s=w80, f="PASS") -> (s? t:f=w122:string)
            n87 = Build Array("\t\tRESULT:", w122) -> (w124:string[])
            n88 = Build Array (concatenate)(w107, w105, w104, w87, w89, w103, w81, w90, w116, w102, w123, w124, w102) -> (w91:string[][])
            n89 = Bundle By Name(cluster=w138, "resultArray2D[]"=w91) -> (w92:T7)
            n90 = Select(t="FAIL", s=w80, f="PASS") -> (s? t:f=w77:string)
            n91 = case shown="\"PASS\"" w77 {
              frame Default {
              }
              frame "FAIL" {
                n92 = call "Read Ini.vi"("key"="Three_colour_Lamp", "section"="Instrument") -> ("error out"=w141:errorcluster, "value"=w140:string)  [unwired: 8 in]
                n93 = call "Control Lamp.vi"("error in (no error)"=w141, "Function Choose"=T8."Reset", "VISA resource name"=w140) -> ("error out"=w148:errorcluster, "VISA resource name out"=w147:refnum<visa-resource-name>)  [unwired: 7 in]
                n94 = call "Control Lamp.vi"("Lamp State"=TRUE, "error in (no error)"=w148, "Function Choose"=T8."Red Lamp&Alarm", "VISA resource name"=w147) -> ()  [unwired: 6 in, 2 out]
              }
              frame "PASS" {
                n95 = call "Read Ini.vi"("key"="Three_colour_Lamp", "section"="Instrument") -> ("error out"=w150:errorcluster, "value"=w149:string)  [unwired: 8 in]
                n96 = call "Control Lamp.vi"("error in (no error)"=w150, "Function Choose"=T8."Reset", "VISA resource name"=w149) -> ("error out"=w157:errorcluster, "VISA resource name out"=w156:refnum<visa-resource-name>)  [unwired: 7 in]
                n97 = call "Control Lamp.vi"("Lamp State"=TRUE, "error in (no error)"=w157, "Function Choose"=T8."Green Lamp&Alarm", "VISA resource name"=w156) -> ()  [unwired: 6 in, 2 out]
              }
            }
          }
          frame "save_log" {
            n98 = Unbundle By Name(w236) -> ("uutInfo.s/n"=w247:string)
            n99 = Unbundle By Name(w242) -> ("userDefind.serverLogPath"=w245:path, "selSeqName"=w243:string)  [unwired: 2 out]
            n100 = Unbundle By Name(w236) -> ("timeStamp.Start"=w239:timestamp, "timeStamp.End"=w240:timestamp)  [unwired: 10 out]
            n101 = Unbundle By Name(w249) -> ("resultArray2D[]"=w241:string[][])
            n102 = Subtract(x=w240, y=w239) -> (x-y=w238:dbl)
            n103 = Number To Fractional String(number=w238, precision (6)=i16 1) -> ()  [unwired: 2 in, 1 out]
            n104 = Array To Spreadsheet String(array=w241, 3:"%s") -> (spreadsheet string=w244:string)  [unwired: 1 in]
            n105 = disable-structure shown="Disabled" {
              disable-tunnel: w247 -> [w285 _]
              disable-tunnel: [w284 _] -> w246
              disable-tunnel: w245 -> [w283 _]
              disable-tunnel: w244 -> [w282 _]
              disable-tunnel: w243 -> [w281 _]
              frame Disabled {
                n106 = Build Path(base path=w283, name or relative path=w281) -> (appended path=w256:path)
                n107 = call <vilib>:"Check if File or Folder Exists.vi"("path"=w256) -> ("error out"=w252:errorcluster, "file or folder exists?"=w255:bool, "dup path"=w254:path)  [unwired: 8 in]
                n108 = case shown="False" w255 {
                  tunnel: w254 -> [w289 w291]
                  tunnel: [w288 w291] -> w253
                  tunnel: w252 -> [w287 w290]
                  tunnel: [w286 w290] -> w251
                  frame False {
                    n109 = Create Folder(path (use dialog)=w289, error in=w287) -> (created path=w288:path, error out=w286:errorcluster)  [unwired: 1 in, 1 out]
                  }
                  frame True {
                  }
                }
                n110 = Concatenate Strings(w285, ".txt" ("string")) -> (w274:string)
                n111 = Concatenate Strings(w285, "H" ("string"), ".txt" ("string")) -> (w271:string)
                n112 = Build Path(base path=w253, name or relative path=w274) -> (appended path=w267:path)
                n113 = Build Path(base path=w253, name or relative path=w271) -> (appended path=w266:path)
                n114 = Open/Create/Replace File(file path (use dialog)=w267, error in=w251, operation (0:open)=T10."replace or create") -> (refnum out=w279:refnum<file>, error out=w277:errorcluster)  [unwired: 3 in, 1 out]
                n115 = Open/Create/Replace File(file path (use dialog)=w266, error in=w251, operation (0:open)=T10."open or create") -> (refnum out=w265:refnum<file>, error out=w264:errorcluster)  [unwired: 3 in, 1 out]
                n116 = Write to Text File(file (use dialog)=w279, text=w282, error in=w277) -> (refnum out=w278:refnum<file>, error out=w276:errorcluster)  [unwired: 1 in, 1 out]
                n117 = Concatenate Strings(w282, "\r\n") -> (w261:string)
                n118 = Set File Position(refnum=w265, from (0:start)=enum16{"start", "end", "current"}."end", error in=w264) -> (refnum out=w263:refnum<file>, error out=w262:errorcluster)  [unwired: 1 in]
                n119 = Write to Text File(file (use dialog)=w263, text=w261, error in=w262) -> (refnum out=w269:refnum<file>, error out=w270:errorcluster)  [unwired: 1 in, 1 out]
                n120 = Close File(refnum=w278, error in=w276) -> (error out=w259:errorcluster)  [unwired: 1 out]
                n121 = Close File(refnum=w269, error in=w270) -> (error out=w258:errorcluster)  [unwired: 1 out]
                n122 = Merge Errors(w259, w258) -> (w284:errorcluster)
              }
              frame Enabled {
              }
            }
          }
          frame "end" {
          }
        }
      }
      frame Error {
      }
    }
  }
  "error out" <- w10
  n123 = Unbundle By Name(w2) -> ("createLogSuccesful"=→"createLogSuccesful":bool)
  "sysVar(Duplicated)" <- "sysVar"
